vi "parseILCModeResponse.vi"(8 "error in (no error)":errorcluster, 10 "DynamicFrameParser":refnum<class "DynamicFrameParser.lvclass">, 11 "ILC in":refnum<class "ILC.lvclass">) -> (0 "error out":errorcluster, 3 "ILC out":refnum<class "ILC.lvclass">)   [LabVIEW 2016, in "RTILC.lvlib" / "ILC.lvclass"]
uses:
  ILC.lvclass
  Common_RT_Modbus/DynamicFrameParser/DynamicFrameParser.lvclass
  Common_RT_Modbus/DataTypes/ExceptionCodes.ctl
  ILC.lvclass/ILC.ctl
  Common_RT_Modbus/RTModbus.lvlib
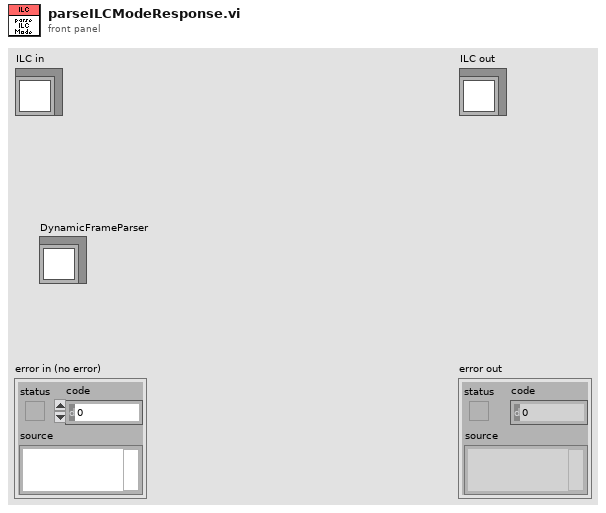
[diagram p1: front panel]
types:
  T1 = typedef "RTModbus.lvlib/ExceptionCodes.ctl" = u16
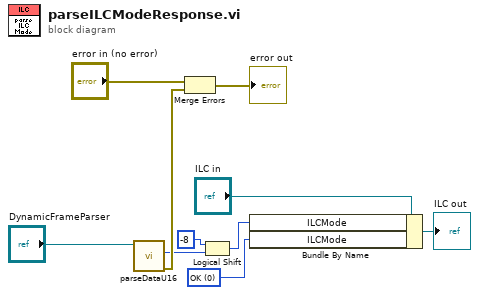
[diagram p0: block diagram]
diagram:
  w4 = T1 0 items=["OK", "IllegalFunction", "IllegalDataAddress", "IllegalDataValue", "SlaveDeviceFailure", "Acknowledge", "SlaveDeviceBusy", "NegativeAcknowledge", "MemoryParityError", "GatewayPathUnavailable", "GatewayTargetDeviceFailedToRespond"] ("ILCData.Responses.ILCMode")
  n1 = call "parseDataU16.vi"("FrameParser in"="DynamicFrameParser") -> ("error out"=w5:errorcluster, "Data"=w3:u16)  [unwired: 8 in, 1 out]
  n2 = Merge Errors("error in (no error)", w5) -> (→"error out":errorcluster)
  n3 = Logical Shift(y=i16 -8, x=w3) -> (x << y=w1:u16)
  n4 = Bundle By Name(cluster="ILC in", "ILCMode"=w1, "ILCMode"=w4) -> (→"ILC out":refnum<class "ILC.lvclass">)
